vi "Add Log File with INI Defaults.vi"(8 "error in":errorcluster, 10 "log file name":string, 11 "embedded data logger in":T1 format="%.0x") -> (0 "error out":errorcluster, 2 "log file":T1 format="%.0x", 3 "embedded data logger out":T1 format="%.0x")   [LabVIEW 2027, in "Embedded Data Logger System Explorer.lvlib"]
uses:
  Embedded Data Logger System Explorer.lvlib
  <vilib>/NI VeriStand/Custom Device API/Custom Device Item Ref.ctl
  Shared/Constants.vi
  Scripting/Embedded Data Logger Scripting.lvlib
  Shared/Embedded Data Logger Shared.lvlib
  <vilib>/NI VeriStand/Custom Device API/Custom Device API.lvlib
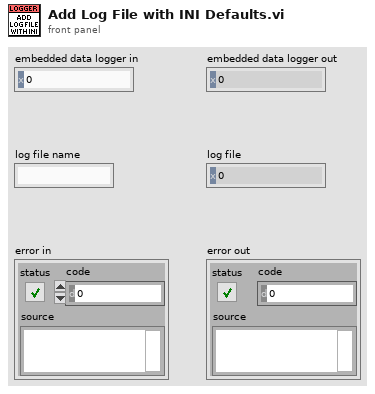
[diagram p1: front panel]
types:
  T1 = typedef "Custom Device API.lvlib/Custom Device Item Ref.ctl" = u64
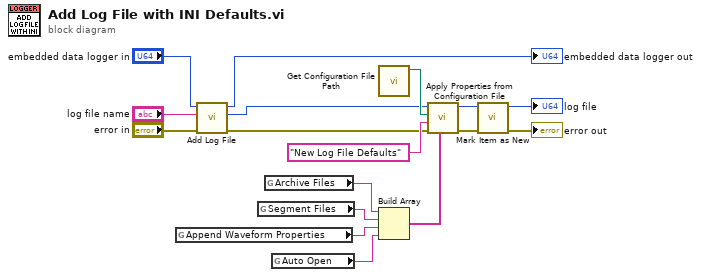
[diagram p0: block diagram]
diagram:
  n1 = global read "Constants.vi" "Append Waveform Properties"() -> (w13:string)
  n2 = call "Add Log File.vi"("error in"="error in", "log file name"="log file name", "embedded data logger in"="embedded data logger in") -> ("error out"=w5:errorcluster, "log file"=w6:T1, "embedded data logger out"=→"embedded data logger out":T1)  [unwired: 6 out]
  n3 = global read "Constants.vi" "Segment Files"() -> (w12:string)
  n4 = global read "Constants.vi" "Archive Files"() -> (w11:string)
  n5 = global read "Constants.vi" "Auto Open"() -> (w1:string)
  n6 = call "Get Configuration File Path.vi"() -> ("Configuration File Path"=w14:path)  [unwired: 11 in]
  n7 = Build Array(w11, w12, w13, w1) -> (w16:string[])
  n8 = call "Apply Properties from Configuration File.vi"("Boolean Properties"=w16, "error in"=w5, "Section"="New Log File Defaults", "Configuration File Path"=w14, "Item Reference In"=w6) -> ("error out"=w15:errorcluster, "Item Device Reference Out"=w3:T1)  [unwired: 5 in]
  n9 = call "Mark Item as New.vi"("error in (no error)"=w15, "Item Ref in"=w3) -> ("error out"=→"error out":errorcluster, "Item Ref out"=→"log file":T1)  [unwired: 8 in]
